vi "event case[1].vi"() -> ()   [LabVIEW 2009]
panel:
  in  "stop":bool
  in  "Test":bool=TRUE
  out "test ok":bool
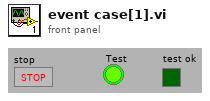
[diagram p1: front panel]
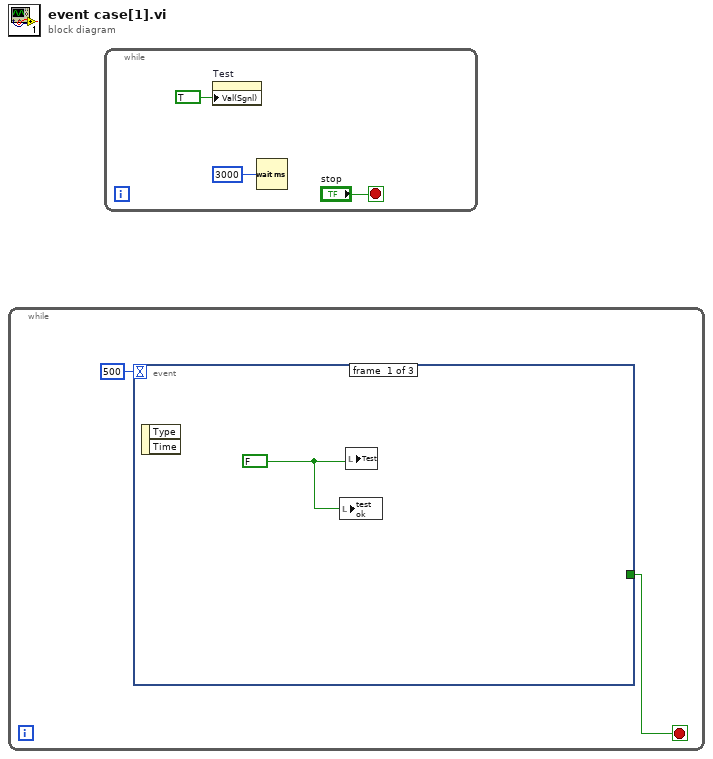
[diagram p0: block diagram]
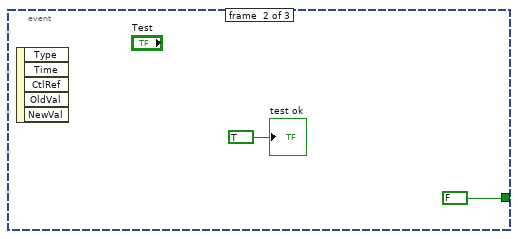
[diagram p2: hidden frame]
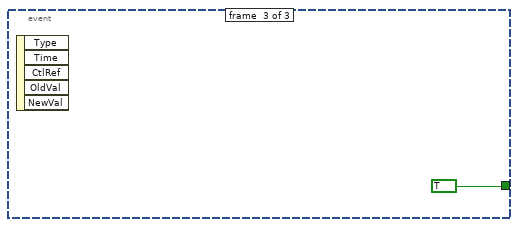
[diagram p3: hidden frame]
diagram:
  n1 = while {
    stop <- w2 stop-if-true
    n2 = event shown="[2] \"stop\": Value Change" {
      selector: _ -> [_ _ _]
      dyn-events: _ -> [_ _ _]
      timeout: 500 -> [_ _ _]
      tunnel: [_ FALSE TRUE] -> w2
      event #0 {
        w3 = FALSE
        n3 = event-data() -> ()  [unwired: 1 in, 2 out]
        n4 = local write "test ok"(w3) -> ()
        n5 = local write "Test"(w3) -> ()
      }
      event #1 {
        n6 = event-data() -> ()  [unwired: 1 in, 5 out]
        "test ok" <- TRUE ("Boolean")
      }
      event #2 {
        n7 = event-data() -> ()  [unwired: 1 in, 5 out]
      }
    }
  }
  n8 = while {
    stop <- "stop" stop-if-true
    n9 = property on="Test" class="Bool (strict)"("Val(Sgnl)"=TRUE ("Value (Signaling)")) -> ()  [unwired: 2 in, 2 out]
    n10 = Wait (ms)(milliseconds to wait=u32 3000 ("Blink Rate")) -> ()  [unwired: 1 out]
  }
